vi "AlliGator Clear Plot(s) Calibration(s).vi"(7 "Phasor Graph Ref":refnum<vi>, 8 "Error In":errorcluster, 9 "Plot Index (-1: last)":i32, 11 "AlliGator IV DVR":refnum<data-value>) -> (0 "Error Out":errorcluster, 1 "Message":string, 2 "# Plots":i32, 3 "AlliGator IV DVR":refnum<data-value>)   [LabVIEW 2021, in "AlliGator Phasor Graph.lvlib"]
doc: "Removes calibration from single, selected or all phasor plots in the Phasor Graph."
uses:
  AlliGator Phasor Graph.lvlib
  AlliGator Internal Variables v2.ctl
  <vilib>/vision/Image Controls.llb/IMAQ Image.ctl
  AlliGator Gate Image Set.ctl
  AlliGator FLI Dataset Type.ctl
  AlliGator Data Series Type.ctl
  AlliGator Dataset Channel.ctl
  AlliGator Gate Arithmetic.ctl
  AlliGator Displayed Image.ctl
  Image/Named ROI Description.ctl
  AlliGator Decay Metadata v3.ctl
  AlliGator Decay Background Subtraction Info.ctl
  AlliGator Baseline Subtraction Method.ctl
  Graphs/XY Graph/XY Graph Plot Shift Parameters.ctl
  Graphs/XY Graph/XY Graph Plot Shift Method.ctl
  AlliGator Decay Extrapolation Parameters.ctl
  Phasor/Calibration Phasor (m, phi).ctl
  Phasor/Phasor Reference Series.ctl
  Phasor/Phasor Calibration Map v2.ctl
  Phasor/Phasor (g, s).ctl
  AlliGator Raw Phasor Plot Data v4.ctl
  Phasor/Phasor Standard Deviation Options.ctl
  AlliGator Phasor Multi-Harmonic Data.ctl
  Phasor/Phasor Harmonic Data.ctl
  AlliGator Decay Fit Options & Parameters v2.ctl
  Fits/IRF(X)PSED/Decay Fit Options v2.ctl
  Fits/Decay Convolution/Decay Model.ctl
  Fits/Residual Type.ctl
  Fits/IRF(X)PSED/Fit Weights Type.ctl
  Fits/Non-linear Fitting Method v2.ctl
  Fits/Fit Calculation Method.ctl
  Fits/Non-linear Fitting Algorithm.ctl
  AlliGator Decay Fit Parameter Constraints 2.ctl
  Fits/IRF(X)PSED/Decay Fit Parameters In List.ctl
  Fits/IRF(X)PSED/MLE Baseline Offset Type.ctl
  AlliGator Decay Preprocessing Parameters.ctl
  Fits/IRF(X)PSED/Decay Fit Parameters & Derived Quantities List.ctl
  Arrays/Arrays.lvlib
  Strings/Strings.lvlib
  Phasor/Phasor.lvlib
  AlliGator Internal Variables.lvlib
  Image/Image.lvlib
  AlliGator Files.lvlib
  AlliGator Decay Preprocessing.lvlib
  Graphs/XY Graph/XY Graph Add-Ons.lvlib
  AlliGator Phasor Plot.lvlib
  AlliGator Source Image.lvlib
  Fits/Fits.lvlib
  AlliGator Decay Fit.lvlib
  AlliGator Decay Fit Parameter Map.lvlib
  AlliGator Settings.lvlib
  AlliGator Dual-Channel Datasets.lvlib
panel:
  # "see the AlliGator License on the block diagram (Ctrl+E or Window:Show Block Diagram)"
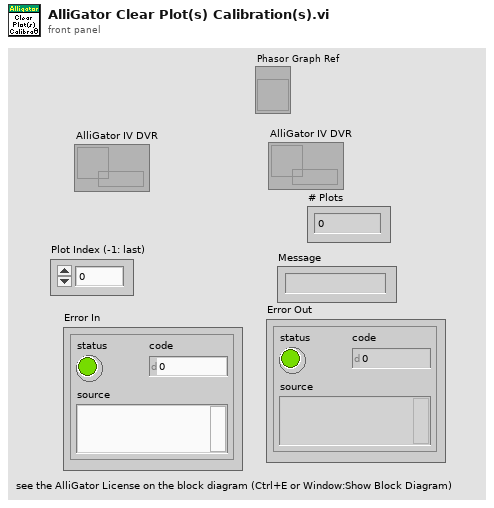
[diagram p1: front panel]
types:
  T1 = typedef "AlliGator Internal Variables.lvlib/AlliGator Internal Variables v2.ctl" = cluster{"Displayed Image":T2, "White Light Image":T2, "Mask Image":T2, "ROI Mask Image":T2, "Current Dataset Images 1":T3, "Background Dataset Images 1":T3, "Current Dataset Images 2":T3, "Background Dataset Images 2":T3, "Current Dataset Arithmetic Images":T3, "Accumulated Dataset Images 1":T3, "Accumulated Dataset Images 2":T3, "Accumulated Dataset Arithmetic Images":T3, "Phasor Plot Image":T2, "Decay Fit Parameter Map Image":T2, "Single Data Point Path":path, "White Light Image Path":path, "Mask Image Path":path, "Time-Series Folder":path, "[Time-Series Paths]":path[], "Current Dataset":i32, "Single Dataset Type":T4, "Current Folder":string, "AlliGator Data Series Type":T5, "# Datasets":i32, "Dual-Channel Dataset":bool, "Selected Channel Name":string, "Dataset Channel":T6, "Channel Arithmetic":T7, "Dual-Channel Background Dataset":bool, "Background Channel":T6, "Dual-Channel Accumulated Dataset":bool, "Start Time":dbl, "[Time-Series Timestamps]":dbl[], "[Intensity Corrections]":dbl[], "Time Series Script":bool, "Type of Displayed Image":T8, "Gate Image Slide":u16, "# Gates":i32, "ROIs":T9[], "ROI Decay":cluster{"t Array":dbl[], "I Array":dbl[]}, "Valid Decay":bool, "Decay  Metadata":T11, "Reference Decay Plot Name":string, "Reference Decay":cluster{"t Array":dbl[], "I Array":dbl[]}, "Decay Shift Plot":cluster{"Time Stamps":dbl[], "Decay Shifts":dbl[]}, "[Decays Max Values]":sgl[], "[Decays Min Values]":sgl[], "Calibration Phasor":T17, "Calibration Phasor Series":T18, "Phasor Calibration Map":T19, "Calibration Map MD5 Digest":string, "Last Raw Phasor":T20, "Last Calibrated Phasor":T20, "Last Calibrated Phasor SDV":T20, "Phasor Graph:Phasor Plot":cluster{"g Array":dbl[], "s Array":dbl[]}, "Phasor Graph:Phasor SDV Plot":cluster{"g Array":dbl[], "s Array":dbl[]}, "[Phasor Graph:Raw Phasor Plots]":T21[], "Phasor Plot locked to Ref 1":i32, "[Phasor Plot(s) locked to Ref 1]":i32[], "[Phasor Plot(s) locked to Ref 2]":i32[], "[Pixel Phasors]":T20[], "[[Sum Image]]":dbl[][], "[[CSG Phasors]]":csg[][], "[[Valid Pixel?]]":bool[][], "I/m/phi Dataset":cluster{"I/m/phi Dataset?":bool, "Base Frequency":dbl[unit], "Harmonic Orders":u8[]}, "Multi Phasor Plot Data":T23, "Decay Fit Options & Parameters":T25, "Fit Options: Decay Preprocessing Parameters":T36, "Fit Options: Reference Decay":cluster{"t Array":dbl[], "I Array":dbl[]}, "Is Full Image Parameters Map":bool, "Is Single-Pixels Parameters Map":bool, "NLSF Parameters Map X Resolution":i32, "NLSF Parameters Map Y Resolution":i32, "[Single Decay Fit Parameters]":dbl[], "Fit Model":T27, "[[Multiple Decays Fit Parameters]]":dbl[][], "[[Multiple Decays Fit Parameter SDVs]]":dbl[][], "[[IRFs]]":dbl[][], "IRF Array Time Axis":dbl[], "Decay Array Time Axis":dbl[], "[Decay Fit Parameter Names]":T37[], "[[Phasor Ratios]]":dbl[][], "[[Average Lifetimes]]":dbl[][], "Amplitude Weighted Average Lifetime":bool, "[Decay Sum]":dbl[], "[[User-defined Quantities]]":dbl[][], "User-defined Quantity":string}
  T2 = typedef "IMAQ Image.ctl" = refnum<image>
  T3 = typedef "AlliGator Files.lvlib/AlliGator Gate Image Set.ctl" = cluster{"SGL Image Max":T2, "SGL Image Sum":T2, "SGL Gate Images":T2[], "SGL Image Min":T2}
  T4 = typedef "AlliGator Files.lvlib/AlliGator FLI Dataset Type.ctl" = enum16{"HDF5 FLI Dataset", "Gate Image Folder", ".sdt FLI Dataset (Becker & Hickl)", ".ptu FLI Dataset (PicoQuant)", "SS1 FLI Dataset", "SS2 FLI Dataset", "I/m/phi Dataset", ".bin FLI Dataset (PicoQuant Binned)", ".bin FLI Dataset (Piccolo Binned)"}
  T5 = typedef "AlliGator Files.lvlib/AlliGator Data Series Type.ctl" = enum16{"Not a Supported Series", "Gate Images Folder Series", "SwissSPAD 2 Dataset Series", "B&H FLI Dataset Series", "PicoQuant PTU FLI Dataset Series", "PicoQuant BIN FLI Dataset Series", "Piccolo hist BIN FLI Dataset Series", "HDF5 FLI Dataset Series"}
  T6 = typedef "AlliGator Dual-Channel Datasets.lvlib/AlliGator Dataset Channel.ctl" = enum16{"G2", "INT"}
  T7 = typedef "AlliGator Settings.lvlib/AlliGator Gate Arithmetic.ctl" = enum16{"None", "INT-G2", "G2/INT*<INT>", "(1 - G2/INT)*<INT>"}
  T8 = typedef "AlliGator Source Image.lvlib/AlliGator Displayed Image.ctl" = enum16{"Single Gate", "Sum of All Gates", "Max of All Gates", "Min of All Gates", "-", "White Ligth Image", "Mask Image"}
  T9 = typedef "Image.lvlib/Named ROI Description.ctl" = cluster{"ROI Descriptor":T10, "ROI Name":string, "Overlay Color":u32}
  T10 = typedef "ROI Descriptor" = cluster{"Global Rectangle":i32[], "Contours":cluster{"ID":enum32{"External", "Internal"}, "Type":u32, "Coordinates":i32[]}[]}
  T11 = typedef "AlliGator Phasor Graph.lvlib/AlliGator Decay Metadata v3.ctl" = cluster{"ROI Descriptor":T10, "ROI Center":cluster{"X":i32, "Y":i32}, "Decay Background Subtraction Info":T12, "Decay Reverted":bool, "Decay Smoothened":bool, "Decay Straightened":bool, "Fitted Tau (Decay Straightening)":dbl, "Decay Shift Parameters":T14, "Decay Shifted":bool, "Decay Extrapolated":bool, "Decay Extrapolation Parameters":T16, "Decay Normalized":bool, "Fold Decay":bool, "# Folds":u32}
  T12 = typedef "AlliGator Decay Analysis.lvlib/AlliGator Decay Preprocessing.lvlib/AlliGator Decay Background Subtraction Info.ctl" = cluster{"Laser Period":dbl[unit], "Gate Duration":dbl[unit], "Baseline Subtraction Method":T13, "Background Definition Range":cluster{"Min Gate":dbl[unit], "Max Gate":dbl[unit]}, "Total Intensity w/o Bkgd Subtraction":dbl, "Bkgd-subtracted Intensity (exp)":dbl, "# Data Points":i32, "Background/Gate":dbl, "Fitted Lifetime":dbl[unit], "Bkgd-subtracted Intensity (theo)":dbl}
  T13 = typedef "AlliGator Decay Analysis.lvlib/AlliGator Decay Preprocessing.lvlib/AlliGator Baseline Subtraction Method.ctl" = enum16{"Mean", "Min", "Square Gated Single-Exponential", "File", "Constant"}
  T14 = typedef "XY Graph Add-Ons.lvlib/XY Graph Plot Shift Parameters.ctl" = cluster{"Type":T15, "Shift":dbl[unit], "Threshold":dbl, "Rotate":bool}
  T15 = typedef "XY Graph Add-Ons.lvlib/XY Graph Plot Shift Method.ctl" = enum16{"Default", "CFD", "Threshold", "Cross-Correlation"}
  T16 = typedef "AlliGator Decay Analysis.lvlib/AlliGator Decay Preprocessing.lvlib/AlliGator Decay Extrapolation Parameters.ctl" = cluster{"Additional Points":u32, "Head Fraction":dbl, "Fitted Tau":dbl, "Use Periodicity":bool, "Use Cursors":bool, "Tail Fraction":dbl}
  T17 = typedef "Phasor.lvlib/Calibration Phasor (m, phi).ctl" = cluster{"m":dbl, "phi":dbl, "Phasor Frequency":dbl[unit], "Reference Lifetime":dbl[unit]}
  T18 = typedef "Phasor.lvlib/Phasor Reference Series.ctl" = cluster{"m Array":dbl[], "phi Array":dbl[], "Phasor Frequency":dbl[unit], "Calibration Lifetime":dbl[unit]}
  T19 = typedef "Phasor.lvlib/Phasor Calibration Map v2.ctl" = cluster{"Phasor Frequency":dbl[unit], "Calibration Lifetime":dbl[unit], "ROI Centers":cluster{"X":i32, "Y":i32}[], "ROI Descriptors":T10[], "Map Resolution X":i32, "Map Resolution Y":i32, "z Array":cdb[]}
  T20 = typedef "Phasor.lvlib/Phasor (g, s).ctl" = cluster{"g":dbl, "s":dbl}
  T21 = typedef "AlliGator Phasor Graph.lvlib/AlliGator Raw Phasor Plot Data v4.ctl" = cluster{"Phasor Plot Name":string, "Raw Phasor Plot":T20[], "Phasor Frequency":dbl[unit], "[Decay Metadata]":T11[], "Raw Phasor Plot SDV":T20[], "Phasor SDV Options":T22, "[Calibration Phasor]":T17[]}
  T22 = typedef "Phasor.lvlib/Phasor Standard Deviation Options.ctl" = cluster{"Compute Estimated SDV":bool, "# Replicas":u32, "Use Estimated Average Phasor":bool}
  T23 = typedef "AlliGator Phasor Plot.lvlib/AlliGator Phasor Multi-Harmonic Data.ctl" = cluster{"Base Frequency":dbl[unit], "# Harmonics":u8, "Harmonic Orders":u8[], "Phasor Plot Settings Checksum":u64, "Phasor Harmonic Data Array":T24[]}
  T24 = typedef "Phasor.lvlib/Phasor Harmonic Data.ctl" = cluster{"Phasor Harmonic Name":string, "Phasor Plot Settings Checksum":u64, "Phasor Frequency":dbl[unit], "Base Frequency":dbl[unit], "Harmonic Order":u8, "Phasor Plot Parameters":string, "Phasor Array [[CSG]]":csg[][], "Dataset File Path":path}
  T25 = typedef "AlliGator Decay Fit Parameter Map.lvlib/AlliGator Decay Fit Options & Parameters v2.ctl" = cluster{"SYNC Period":dbl[unit], "Fit Options":T26, "Fit Parameter Constraints":T33[], "MLE Baseline Offset":dbl, "MLE Baseline Offset Type":T35}
  T26 = typedef "Fits.lvlib/Decay Fit Options v2.ctl" = cluster{"Show Fit Residuals":bool, "Fit Model":T27, "Residual Type":T28, "Max Decay Percentile":dbl, "Min Decay Percentile":dbl, "Show Full Decay":bool, "Weights":T29, "Fitting Method":T30, "Compute Parameter Uncertainties":bool, "Periodic Boundaries":bool, "Model Calculation":T31, "Period":dbl[unit], "Termination Criteria":cluster{"Max Iterations":i32, "Max Function Calls":i32, "Max Time":dbl[unit], "Function Tolerance":dbl, "Parameter Tolerance":dbl, "Gradient Tolerance":dbl, "Min Lambda":dbl, "Max Lambda":dbl, "Initial Tick Count":u32}, "Offset Resolution":dbl[unit], "Use Local IRF":bool, "Fitting Algorithm":T32}
  T27 = typedef "Fits.lvlib/Decay Model.ctl" = enum16{"1-Exponential", "2-Exponentials"}
  T28 = typedef "Fits.lvlib/Residual Type.ctl" = enum16{"Standard", "Normalized", "Reduced"}
  T29 = typedef "Fits.lvlib/Fit Weights Type.ctl" = enum16{"Unweighted", "1/Variance", "Best of All"}
  T30 = typedef "Fits.lvlib/Non-linear Fitting Method v2.ctl" = enum16{"Least Square", "Least Absolute Residual", "Bisquare", "MLE", "-", "Best of All"}
  T31 = typedef "Fits.lvlib/Fit Calculation Method.ctl" = enum16{"Simulation", "Convolution", "Integration"}
  T32 = typedef "Fits.lvlib/Non-linear Fitting Algorithm.ctl" = enum16{"Levenberg-Marquardt", "Trust-Region Dogleg"}
  T33 = typedef "AlliGator Decay Analysis.lvlib/AlliGator Decay Fit.lvlib/AlliGator Decay Fit Parameter Constraints 2.ctl" = cluster{"Fit Parameter":T34, "Min Value":dbl, "Max Value":dbl, "Global":bool, "Used":bool}
  T34 = typedef "Fits.lvlib/Decay Fit Parameters In List.ctl" = enum16{"Offset", "Baseline", "A_1", "tau_1", "A_2", "tau_2"}
  T35 = typedef "Fits.lvlib/MLE Baseline Offset Type.ctl" = enum32{"Absolute", "Percentage"}
  T36 = typedef "AlliGator Decay Analysis.lvlib/AlliGator Decay Preprocessing.lvlib/AlliGator Decay Preprocessing Parameters.ctl" = cluster{"Background Subtraction":bool, "Straighten Decay":bool, "Reverse Gates":bool, "1-Normalized Decay":bool, "Smoothen Decay":bool, "Smoothing Parameter":dbl, "Shift Decay":bool, "Decay Shift Parameters":T14, "Extrapolate Decay":bool, "Additional Points":u32, "Head Fraction":dbl, "Pixel-Normalize Decay":bool, "Use Periodicity":bool, "Use Cursors":bool, "Tail Fraction":dbl, "Use Decay Pre-Processing":bool, "Fold Decay":bool, "# Folds":u32, "[0-1]-Normalized Decay":bool}
  T37 = typedef "Fits.lvlib/Decay Fit Parameters & Derived Quantities List.ctl" = enum16{"Offset", "Baseline", "A_1", "tau_1", "A_2", "tau_2", "<tau>_a", "f1_a", "f2_a", "<tau>_i", "f1_i", "f2_i", "-", "R^2", "Chi^2"}
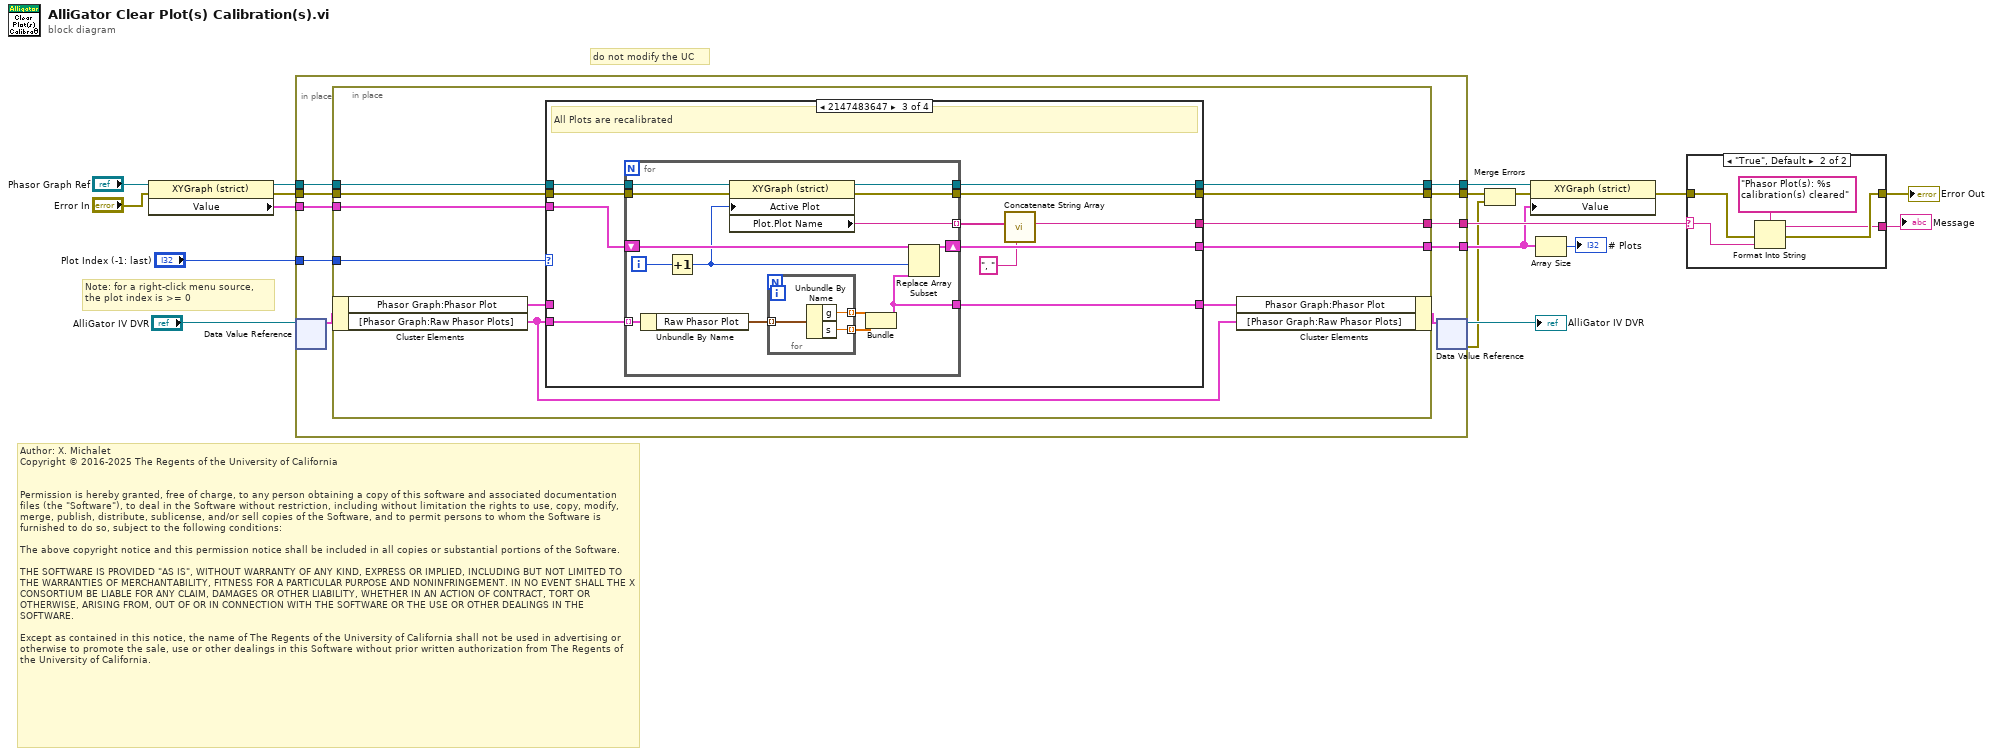
[diagram p0: block diagram]
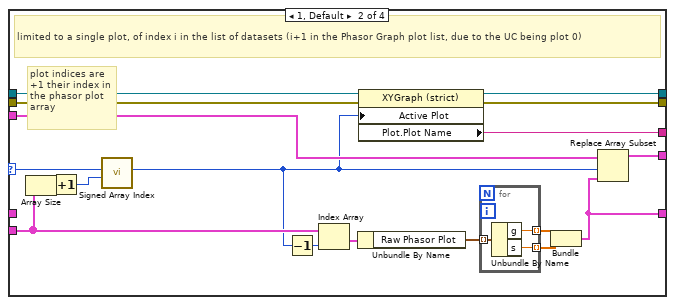
[diagram p4: hidden frame]
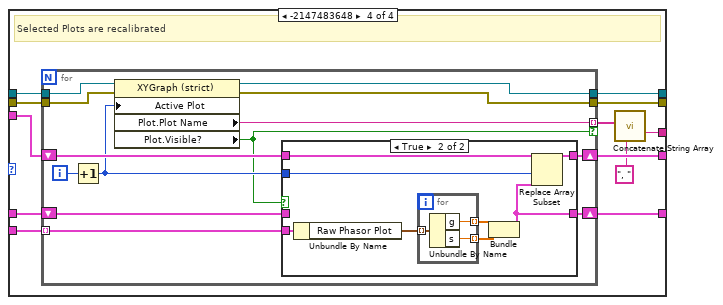
[diagram p5: hidden frame]
diagram:
  # "Author: X. Michalet\nCopyright © 2016-2025 The Regents of the University of California\n \n\nPermission is hereby granted, free of charge, to any person obtaining a copy of this software and associated documentation files (the \"Software\"), to deal in the Software without restriction, including without limitation the rights to use, copy, modify, merge, publish, distribute, sublicense, and/or sell copies of the Software, and to permit persons to whom the Software is furnished to do so, subject to the following conditions:\n\nThe above copyright notice and this permission notice shall be included in all copies or substantial portions of the Software.\n\nTHE SOFTWARE IS PROVIDED \"AS IS\", WITHOUT WARRANTY OF ANY KIND, EXPRESS OR IMPLIED, INCLUDING BUT NOT LIMITED TO THE WARRANTIES OF MERCHANTABILITY, FITNESS FOR A PARTICULAR PURPOSE AND NONINFRINGEMENT. IN NO EVENT SHALL THE X CONSORTIUM BE LIABLE FOR ANY CLAIM, DAMAGES OR OTHER LIABILITY, WHETHER IN AN ACTION OF CONTRACT, TORT OR OTHERWISE, ARISING FROM, OUT OF OR IN CONNECTION WITH THE SOFTWARE OR THE USE OR OTHER DEALINGS IN THE SOFTWARE.\n\nExcept as contained in this notice, the name of The Regents of the University of California shall not be used in advertising or otherwise to promote the sale, use or other dealings in this Software without prior written authorization from The Regents of the University of California."
  # "Note: for a right-click menu source,\nthe plot index is >= 0"
  # "do not modify the UC"
  n1 = property class="XYGraph (strict)"(reference="Phasor Graph Ref", error in="Error In") -> (reference out=w12:refnum<vi>, error out=w9:errorcluster, "Value"=w13:cluster{"X Array":dbl[], "Y Array":dbl[]}[])
  n2 = in-place {
    in-place-border: "Plot Index (-1: last)" -> [w26]
    in-place-border: w13 -> [w25]
    in-place-border: [w24] -> w7
    in-place-border: w12 -> [w23]
    in-place-border: [w22] -> w10
    in-place-border: [w21] -> w11
    in-place-border: w9 -> [w20]
    in-place-border: [w19] -> w8
    n3 = in-place-dvr #1("AlliGator IV DVR") -> (w28:T1)  [unwired: 1 out]
    n4 = in-place {
      in-place-border: w26 -> [w39]
      in-place-border: w25 -> [w38]
      in-place-border: [w37] -> w24
      in-place-border: w23 -> [w35]
      in-place-border: [w34] -> w22
      in-place-border: [w33] -> w21
      in-place-border: w20 -> [w32]
      in-place-border: [w31] -> w19
      n5 = in-place-cluster #2(w28) -> ("Phasor Graph:Phasor Plot"=w30:cluster{"g Array":dbl[], "s Array":dbl[]}, "[Phasor Graph:Raw Phasor Plots]"=w36:T21[])
      n6 = case shown="2147483647" w39 {
        selector: w39 -> [_ w51 _ _]
        tunnel: w36 -> [_ w58 w74 w103]
        tunnel: w38 -> [w41 w60 w75 w104]
        tunnel: [w41 w59 w73 w102] -> w37
        tunnel: w35 -> [w43 w57 w72 w101]
        tunnel: [_ w54 w69 w98] -> w34
        tunnel: [w43 w55 w71 w100] -> w33
        tunnel: w32 -> [w42 w53 w67 w96]
        tunnel: [w42 w52 w66 w95] -> w31
        tunnel: w30 -> [w40 _ _ w93]
        tunnel: [w40 w50 w65 w94] -> w29
        frame 0 {
          # "UC: do nothing"
        }
        frame 1, Default {
          # "plot indices are\n+1 their index in the phasor plot array"
          # "limited to a single plot, of index i in the list of datasets (i+1 in the Phasor Graph plot list, due to the UC being plot 0)"
          n7 = Array Size(array=w58) -> (size(s)=w61:i32)
          n8 = Increment(x=w61) -> (x+1=w49:i32)
          n9 = call "Signed Array Index.vi"("Array Size"=w49, "Array Index in"=w51) -> ("Array Index out"=w56:i32)  [unwired: 9 in]
          n10 = Decrement(x=w56) -> (x-1=w47:i32)
          n11 = Index Array(array=w58, index=w47) -> (element=w48:T21)
          n12 = Unbundle By Name(w48) -> ("Raw Phasor Plot"=w46:T20[])
          n13 = property class="XYGraph (strict)"(reference=w57, error in=w53, "Active Plot"=w56) -> (reference out=w55:refnum<vi>, error out=w52:errorcluster, "Plot.Plot Name"=w54:string)
          n14 = for {
            tunnel: w46 -> [w64] mode=indexing
            tunnel: [w63] -> w45 mode=indexing
            tunnel: [w62] -> w44 mode=indexing
            n15 = Unbundle By Name(w64) -> ("g"=w63:dbl, "s"=w62:dbl)
          }
          n16 = Bundle(w45, w44) -> (w50:cluster{dbl[], dbl[]})  [unwired: 1 in]
          n17 = Replace Array Subset(array=w60, new element=w50, index=w56) -> (w59:cluster{"X Array":dbl[], "Y Array":dbl[]}[])
        }
        frame 2147483647 {
          # "All Plots are recalibrated"
          n18 = for {
            shift-right: [w88] -> w73
            shift-left: w75 -> [w89]
            tunnel: w74 -> [w87] mode=indexing
            tunnel: w72 -> [w86]
            tunnel: [w85] -> w71
            tunnel: [w84] -> w70 mode=indexing
            tunnel: w67 -> [w83]
            tunnel: [w82] -> w66
            tunnel: [w76] -> w65
            i -> [w81]
            n19 = Unbundle By Name(w87) -> ("Raw Phasor Plot"=w77:T20[])
            n20 = Increment(x=w81) -> (x+1=w80:i32)
            n21 = property class="XYGraph (strict)"(reference=w86, error in=w83, "Active Plot"=w80) -> (reference out=w85:refnum<vi>, error out=w82:errorcluster, "Plot.Plot Name"=w84:string)
            n22 = for {
              tunnel: w77 -> [w92] mode=indexing
              tunnel: [w91] -> w79 mode=indexing
              tunnel: [w90] -> w78 mode=indexing
              n23 = Unbundle By Name(w92) -> ("g"=w91:dbl, "s"=w90:dbl)
            }
            n24 = Bundle(w79, w78) -> (w76:cluster{dbl[], dbl[]})  [unwired: 1 in]
            n25 = Replace Array Subset(array=w89, new element=w76, index=w80) -> (w88:cluster{"X Array":dbl[], "Y Array":dbl[]}[])
          }
          n26 = call "Concatenate String Array.vi"("Separator (TAB)"=", ", "String Array"=w70) -> ("Formatted String"=w69:string)  [unwired: 9 in]
        }
        frame -2147483648 {
          # "Selected Plots are recalibrated"
          n27 = for {
            shift-right: [w116] -> w102
            shift-left: w104 -> [w117]
            tunnel: w103 -> [w115] mode=indexing
            tunnel: w101 -> [w114]
            tunnel: [w113] -> w100
            tunnel: [w112] -> w99 mode=indexing if=w106
            tunnel: w96 -> [w111]
            tunnel: [w110] -> w95
            shift-right: [w107] -> w94
            shift-left: w93 -> [w105]
            i -> [w109]
            n28 = Increment(x=w109) -> (x+1=w108:i32)
            n29 = property class="XYGraph (strict)"(reference=w114, error in=w111, "Active Plot"=w108) -> (reference out=w113:refnum<vi>, error out=w110:errorcluster, "Plot.Plot Name"=w112:string, "Plot.Visible?"=w106:bool)
            n30 = case shown="True" w106 {
              tunnel: w117 -> [w119 w127]
              tunnel: [w119 w126] -> w116
              tunnel: w115 -> [_ w125]
              tunnel: w108 -> [_ w124]
              tunnel: [w118 w120] -> w107
              tunnel: w105 -> [w118 _]
              frame False {
              }
              frame True {
                n31 = Unbundle By Name(w125) -> ("Raw Phasor Plot"=w121:T20[])
                n32 = for {
                  tunnel: w121 -> [w130] mode=indexing
                  tunnel: [w129] -> w123 mode=indexing
                  tunnel: [w128] -> w122 mode=indexing
                  n33 = Unbundle By Name(w130) -> ("g"=w129:dbl, "s"=w128:dbl)
                }
                n34 = Bundle(w123, w122) -> (w120:cluster{dbl[], dbl[]})  [unwired: 1 in]
                n35 = Replace Array Subset(array=w127, new element=w120, index=w124) -> (w126:cluster{"X Array":dbl[], "Y Array":dbl[]}[])
              }
            }
          }
          n36 = call "Concatenate String Array.vi"("Separator (TAB)"=", ", "String Array"=w99) -> ("Formatted String"=w98:string)  [unwired: 9 in]
        }
      }
      n37 = in-place-cluster #2("Phasor Graph:Phasor Plot"=w29, "[Phasor Graph:Raw Phasor Plots]"=w36) -> (w27:T1)
    }
    n38 = in-place-dvr #1(w27) -> (→"AlliGator IV DVR":refnum<data-value>, w3:errorcluster)
  }
  n39 = Merge Errors(w8, w3) -> (w4:errorcluster)
  n40 = property class="XYGraph (strict)"(reference=w11, error in=w4, "Value"=w7) -> (error out=w5:errorcluster)  [unwired: 1 out]
  n41 = Array Size(array=w7) -> (size(s)=→"# Plots":i32)
  n42 = case shown="\"True\", Default" w10 {
    selector: w10 -> [_ w135]
    tunnel: w5 -> [w131 w134]
    tunnel: [w131 w133] -> w2
    tunnel: [_ w132] -> w1
    frame "" {
    }
    frame "True", Default {
      n43 = Format Into String(format string="Phasor Plot(s): %s calibration(s) cleared", error in=w134, w135) -> (resulting string=w132:string, error out=w133:errorcluster)  [unwired: 1 in]
    }
  }
  "Error Out" <- w2
  "Message" <- w1
